vi "Byte Array to Hex String Conversion.vi"(8 "Error In":errorcluster, 11 "Array":u8[](array[numeric])) -> (0 "Error Out":errorcluster, 3 "String":string)   [LabVIEW 2018, in "Hitronics.lvlib" / "Hitronics.lvclass"]
uses:
  Hitronics.lvclass
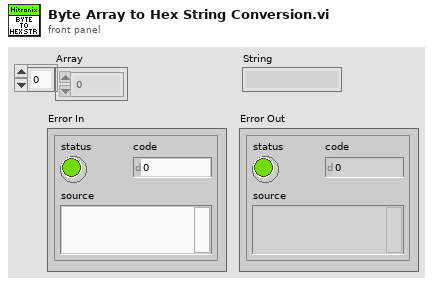
[diagram p1: front panel]
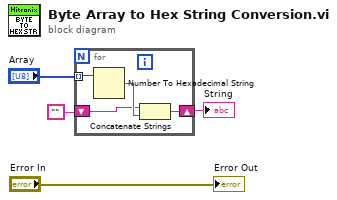
[diagram p0: block diagram]
diagram:
  n1 = for {
    tunnel: "Array" -> [w8] mode=indexing
    shift-right: [w5] -> w2
    shift-left: "" -> [w6]
    n2 = Number To Hexadecimal String(2:w8) -> (0:w7:string)  [unwired: 1 in]
    n3 = Concatenate Strings(w6, w7) -> (w5:string)
  }
  "String" <- w2
  "Error Out" <- "Error In"
